vi "ProdaNG.Tree.Delete.vi"(7 "TestStepsTree":refnum<vi>, 8 "error in (no error)":errorcluster, 10 "Elements to delete":T1[](array[typedef]), 11 "dbHandleIn":i32) -> (0 "error out":errorcluster, 3 "dbHandle":i32)   [LabVIEW 2016]
uses:
  ProdaNG.Tree.Fglb.Data.ctl
  ProdaNG.Tree.Fglb.Element.ctl
  ProdaNG.Configurator.Glb.vi
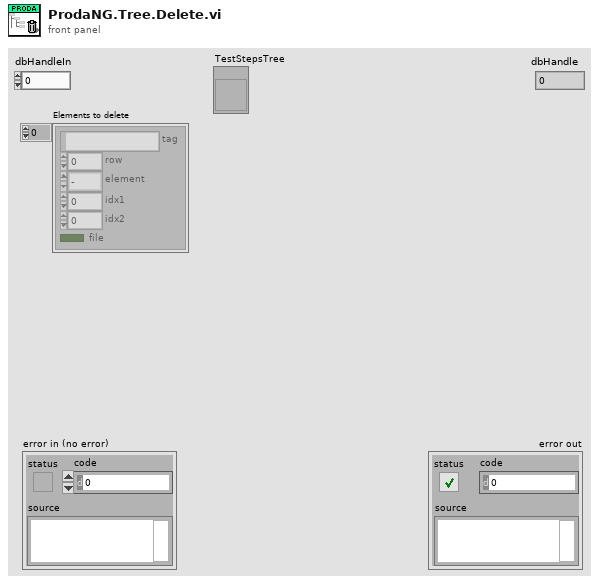
[diagram p1: front panel]
types:
  T1 = typedef "ProdaNG.Tree.Fglb.Data.ctl" = cluster{"tag":string, "row":i32, "element":T2, "idx1":i32, "idx2":i32, "file":bool}
  T2 = typedef "ProdaNG.Tree.Fglb.Element.ctl" = enum16{"-", "PP", "TS", "TP", "TV"}
  T3 = typedef "ProdaNG.ProcessStepParam.ctl" = cluster{"i_id":i32, "processStepId":i32, "unitId":i32, "contentId":string, "previewId":string, "value":dbl, "valueText":string, "paramSequence":i32, "history":i32, "mdReason":string, "mdUser":string, "mdTime":string, "description":string}
  T4 = typedef "ProdaNG.TestStep.ctl" = cluster{"i_id":i32, "processStepId":i32, "testSequence":i32, "testOrder":i32, "mdReason":string, "mdUser":string, "mdTime":string, "description":string}
  T5 = typedef "ProdaNG.TestStepParam.ctl" = cluster{"i_id":i32, "testStepId":i32, "unitId":i32, "contentId":string, "previewId":string, "value":dbl, "valueText":string, "paramSequence":i32, "history":i32, "mdReason":string, "mdUser":string, "mdTime":string, "description":string}
  T6 = typedef "ProdaNG.TestValue.ctl" = cluster{"i_id":i32, "testStepId":i32, "releaseId":i32, "unitId":i32, "contentId":string, "previewId":string, "maximum":dbl, "minimum":dbl, "valueText":string, "testValueSequence":i32, "history":i32, "mdReason":string, "mdUser":string, "mdTime":string, "description":string}
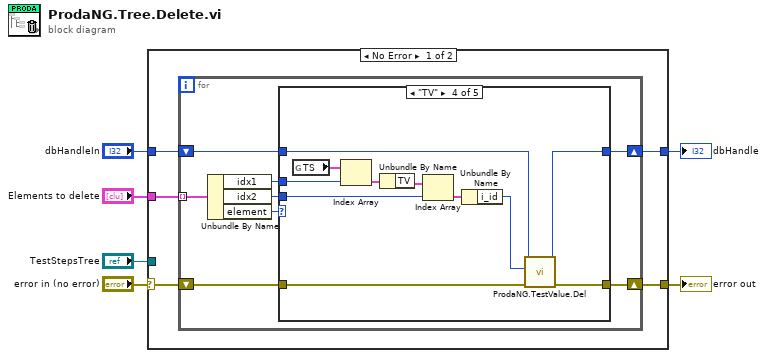
[diagram p0: block diagram]
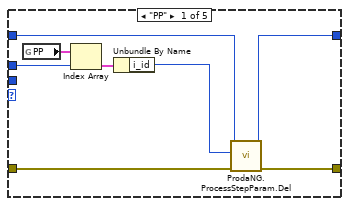
[diagram p2: hidden frame]
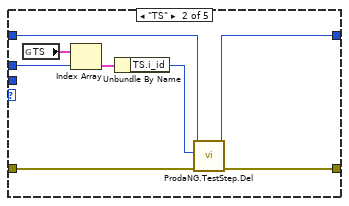
[diagram p3: hidden frame]
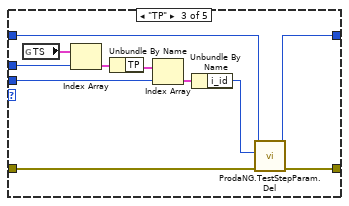
[diagram p4: hidden frame]
diagram:
  n1 = case shown="No Error" "error in (no error)" {
    selector: "error in (no error)" -> [w7 w61]
    tunnel: "TestStepsTree" -> [_ _]
    tunnel: [w11 w61] -> w6
    tunnel: "dbHandleIn" -> [w10 w60]
    tunnel: [w9 w60] -> w2
    tunnel: "Elements to delete" -> [w8 _]
    frame No Error {
      n2 = for {
        shift-right: [w17] -> w11
        shift-left: w7 -> [w13]
        shift-right: [w15] -> w9
        shift-left: w10 -> [w16]
        tunnel: w8 -> [w14] mode=indexing
        n3 = Unbundle By Name(w14) -> ("idx1"=w18:i32, "idx2"=w12:i32, "element"=w19:T2)
        n4 = case shown="\"TV\"" w19 {
          tunnel: w18 -> [w27 w35 w46 w57 _]
          tunnel: w13 -> [w22 w33 w37 w48 w59]
          tunnel: [w25 w32 w44 w55 w59] -> w17
          tunnel: w16 -> [w24 w31 w43 w54 w58]
          tunnel: [w23 w30 w42 w53 w58] -> w15
          tunnel: w12 -> [_ _ w40 w51 _]
          frame "PP" {
            n5 = global read "ProdaNG.Configurator.Glb.vi" "PP"() -> (w26:T3[])
            n6 = Index Array(array=w26, index=w27) -> (element=w21:T3)
            n7 = Unbundle By Name(w21) -> ("i_id"=w20:i32)
            n8 = call "ProdaNG.ProcessStepParam.Del.vi"("error in (no error)"=w22, "ProcessStepParamId"=w20, "dbHandleIn"=w24) -> ("error out"=w25:errorcluster, "dbHandle"=w23:i32)  [unwired: 7 in]
          }
          frame "TS" {
            n9 = global read "ProdaNG.Configurator.Glb.vi" "TS"() -> (w34:cluster{"TS":T4, "TP":T5[], "TV":T6[]}[])
            n10 = Index Array(array=w34, index=w35) -> (element=w29:cluster{"TS":T4, "TP":T5[], "TV":T6[]})
            n11 = Unbundle By Name(w29) -> ("TS.i_id"=w28:i32)
            n12 = call "ProdaNG.TestStep.Del.vi"("error in (no error)"=w33, "TestStepId"=w28, "dbHandleIn"=w31) -> ("error out"=w32:errorcluster, "dbHandle"=w30:i32)  [unwired: 7 in]
          }
          frame "TP" {
            n13 = global read "ProdaNG.Configurator.Glb.vi" "TS"() -> (w45:cluster{"TS":T4, "TP":T5[], "TV":T6[]}[])
            n14 = Index Array(array=w45, index=w46) -> (element=w41:cluster{"TS":T4, "TP":T5[], "TV":T6[]})
            n15 = Unbundle By Name(w41) -> ("TP"=w39:T5[])
            n16 = Index Array(array=w39, index=w40) -> (element=w38:T5)
            n17 = Unbundle By Name(w38) -> ("i_id"=w36:i32)
            n18 = call "ProdaNG.TestStepParam.Del.vi"("error in (no error)"=w37, "TestStepParamId"=w36, "dbHandleIn"=w43) -> ("error out"=w44:errorcluster, "dbHandle"=w42:i32)  [unwired: 7 in]
          }
          frame "TV" {
            n19 = global read "ProdaNG.Configurator.Glb.vi" "TS"() -> (w56:cluster{"TS":T4, "TP":T5[], "TV":T6[]}[])
            n20 = Index Array(array=w56, index=w57) -> (element=w52:cluster{"TS":T4, "TP":T5[], "TV":T6[]})
            n21 = Unbundle By Name(w52) -> ("TV"=w50:T6[])
            n22 = Index Array(array=w50, index=w51) -> (element=w49:T6)
            n23 = Unbundle By Name(w49) -> ("i_id"=w47:i32)
            n24 = call "ProdaNG.TestValue.Del.vi"("error in (no error)"=w48, "TestStepId"=w47, "dbHandleIn"=w54) -> ("error out"=w55:errorcluster, "dbHandle"=w53:i32)  [unwired: 7 in]
          }
          frame Default {
          }
        }
      }
    }
    frame Error {
    }
  }
  "error out" <- w6
  "dbHandle" <- w2
